vi "GlyphIndexPairs.vi"(7 "enum":T1, 9 "array":T2[](array[typedef]), 10 "glyph":string) -> (2 "index":i32)   [LabVIEW 2013, in "NISE_CEF_TreeControl.lvlib"]
uses:
  NISE_CEF_TreeControl.lvlib
  Controls/GlyphIndexPair.ctl
  Controls/GlyphIndexPairActions.ctl
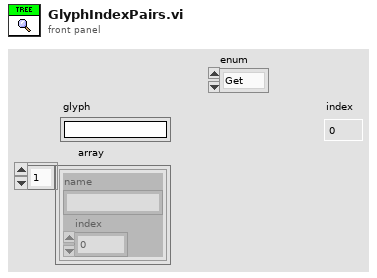
[diagram p1: front panel]
types:
  T1 = typedef "NISE_CEF_TreeControl.lvlib/GlyphIndexPairActions.ctl" = enum16{"Get", "Initialize"}
  T2 = typedef "NISE_CEF_TreeControl.lvlib/GlyphIndexPair.ctl" = cluster{"name":string, "index":i32}
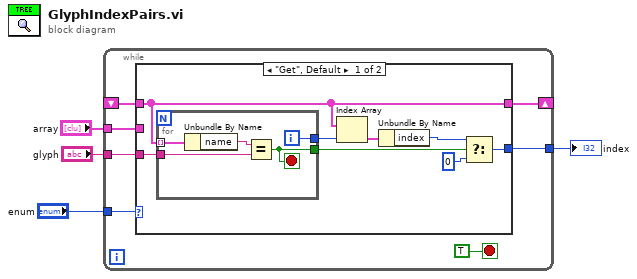
[diagram p0: block diagram]
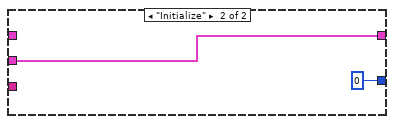
[diagram p2: hidden frame]
diagram:
  n1 = while {
    tunnel: "glyph" -> [w11]
    tunnel: [w10] -> w3
    shift-right: [w7] -> _
    shift-left: _ -> [w8]
    tunnel: "array" -> [w6]
    tunnel: "enum" -> [w5]
    stop <- TRUE stop-if-true
    n2 = case shown="\"Get\", Default" w5 {
      tunnel: w11 -> [w19 _]
      tunnel: [w14 0 ("f")] -> w10
      tunnel: w8 -> [w12 _]
      tunnel: [w12 w25] -> w7
      tunnel: w6 -> [_ w25]
      frame "Get", Default {
        n3 = for {
          tunnel: w12 -> [w24] mode=indexing
          tunnel: w19 -> [w23]
          tunnel: [w21] -> w17
          tunnel: [w20] -> w18
          i -> [w21]
          stop <- w20 stop-if-true
          n4 = Unbundle By Name(w24) -> ("name"=w22:string)
          n5 = Equal?(x=w22, y=w23) -> (x = y?=w20:bool)
        }
        n6 = Index Array(array=w12, index=w17) -> (element=w13:T2)
        n7 = Unbundle By Name(w13) -> ("index"=w16:i32)
        n8 = Select(t=w16, s=w18, f=0) -> (s? t:f=w14:i32)
      }
      frame "Initialize" {
      }
    }
  }
  "index" <- w3
